vi "DataBuffer.vi"(0 "Enum":enum16{"Maintain", "Update", "Initialise"}(ring), 1 "Current (A) In":dbl, 2 "Magnet Current (A) In":dbl, 3 "Voltage (V) In":dbl, 4 "Switch Htr State In":bool) -> (15 "Current (A) Out":dbl, 16 "Magnet Current (A) Out":dbl, 17 "Voltage (V) Out":dbl, 18 "Sw Htr State Out":bool)   [LabVIEW 2019]
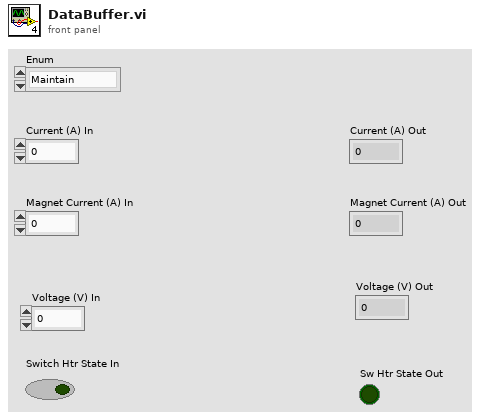
[diagram p1: front panel]
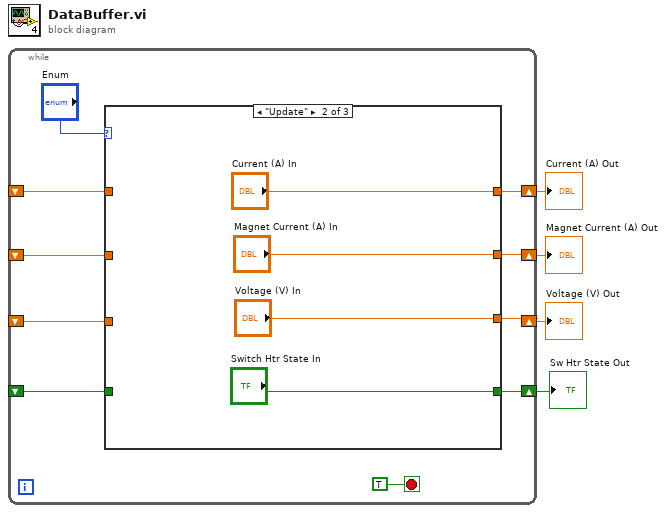
[diagram p0: block diagram]
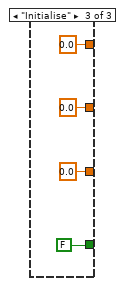
[diagram p3: hidden frame]
diagram:
  n1 = while {
    shift-right: [w10] -> w4
    shift-left: _ -> [w9]
    shift-right: [w11] -> w3
    shift-left: _ -> [w8]
    shift-right: [w12] -> w2
    shift-left: _ -> [w7]
    shift-right: [w6] -> w1
    shift-left: _ -> [w5]
    stop <- TRUE stop-if-true
    n2 = case shown="\"Update\"" "Enum" {
      tunnel: [w18 "Current (A) In" 0.0 ("Current (A)")] -> w10
      tunnel: [w17 "Magnet Current (A) In" 0.0 ("Magnet Current (A)")] -> w11
      tunnel: [w16 "Voltage (V) In" 0.0 ("Voltage (V)")] -> w12
      tunnel: w9 -> [w18 _ _]
      tunnel: w8 -> [w17 _ _]
      tunnel: w7 -> [w16 _ _]
      tunnel: [w15 "Switch Htr State In" FALSE] -> w6
      tunnel: w5 -> [w15 _ _]
      frame "Maintain", Default {
      }
      frame "Update" {
      }
      frame "Initialise" {
      }
    }
  }
  "Current (A) Out" <- w4
  "Magnet Current (A) Out" <- w3
  "Voltage (V) Out" <- w2
  "Sw Htr State Out" <- w1
